vi "DAQ_Torque_Cell.vi"(6 "stop 2":bool) -> ()   [LabVIEW 2020]
doc: "I. Description:\nThis example demonstrates how to continuously acquire data (Waveform) using the DAQ device's internal clock and an analog slope start trigger.\n\nII. Instructions for Running:\n1. Select the physical channel to correspond to where your signal is input on the DAQ device.\n2. Enter the minimum and maximum voltage ranges.\nNote: For better accuracy try to match the Input Ranges to the expected voltage level of the measured signal.\n3. Set the rate of the acquisition. Also set the Samples to Read control. This will determine how many samples are read each time the while loop iterates. This also determines how many points are plotted on the graph each iteration.\nNote: The rate should be at least twice as fast as the maximum frequency component of the signal being acquired.\n4. Set the source of the Analog Slope Start Trigger.\n5. Set the slope and level of desired analog edge condition.\n\nIII. Block Diagram Steps:\n1. Create an analog input voltage channel.\n2. Set the rate for the sample clock. Additionally, define the sample mode to be continuous.\n3. Define the parameters for an Analog Slope Start Trigger.\n4. Call the Start VI to start the acquisition.\n5. Read the waveform data in a loop until the user hits the stop button or an error occurs.\n6. Call the Clear Task VI to clear the Task.\n7. Use the popup dialog box to display an error if any.\n\nIV. I/O Connections Overview:\nMake sure your signal input terminal matches the Physical Channel I/O control. Also, make sure your analog trigger terminal matches the Trigger Source Control. For further connection information, refer to your hardware reference manual."
uses:
  <vilib>/Utility/error.llb/DialogType.ctl
  <vilib>/ULx/Create Channel.llb/ULx Create Channel (AI-Voltage-Basic).vi
  <vilib>/ULx/Timing.llb/ULx Timing (Sample Clock).vi
  <vilib>/ULx/Read.llb/ULx Read (Analog Wfm 1Chan NSamp).vi
panel:
  out "Torque Graph":waveform(dbl)(graph)
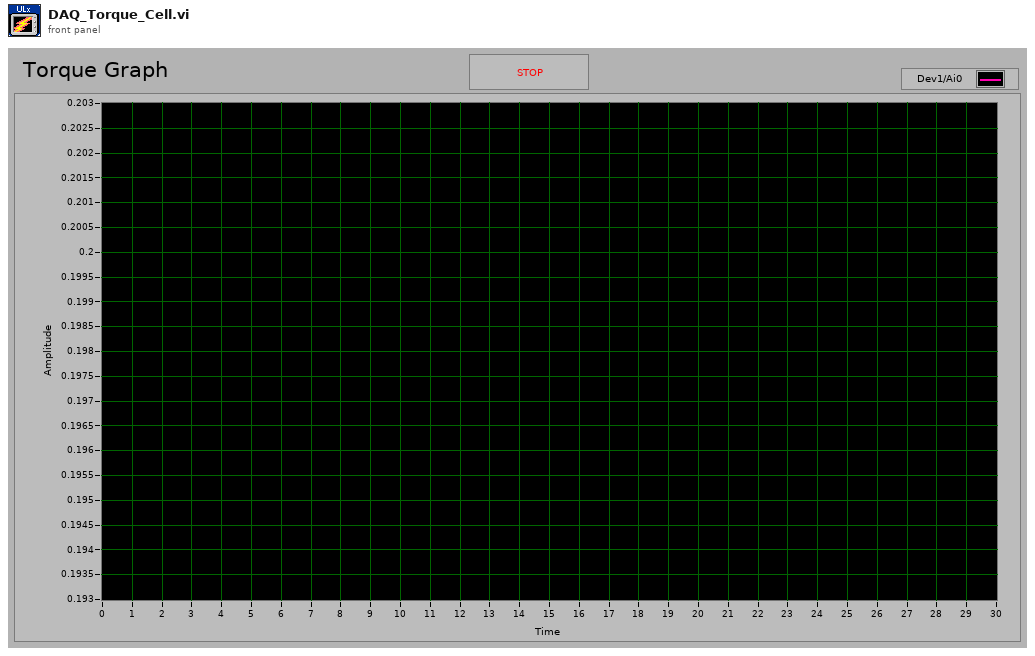
[diagram p1: front panel]
types:
  T1 = typedef "DialogType.ctl" = u16
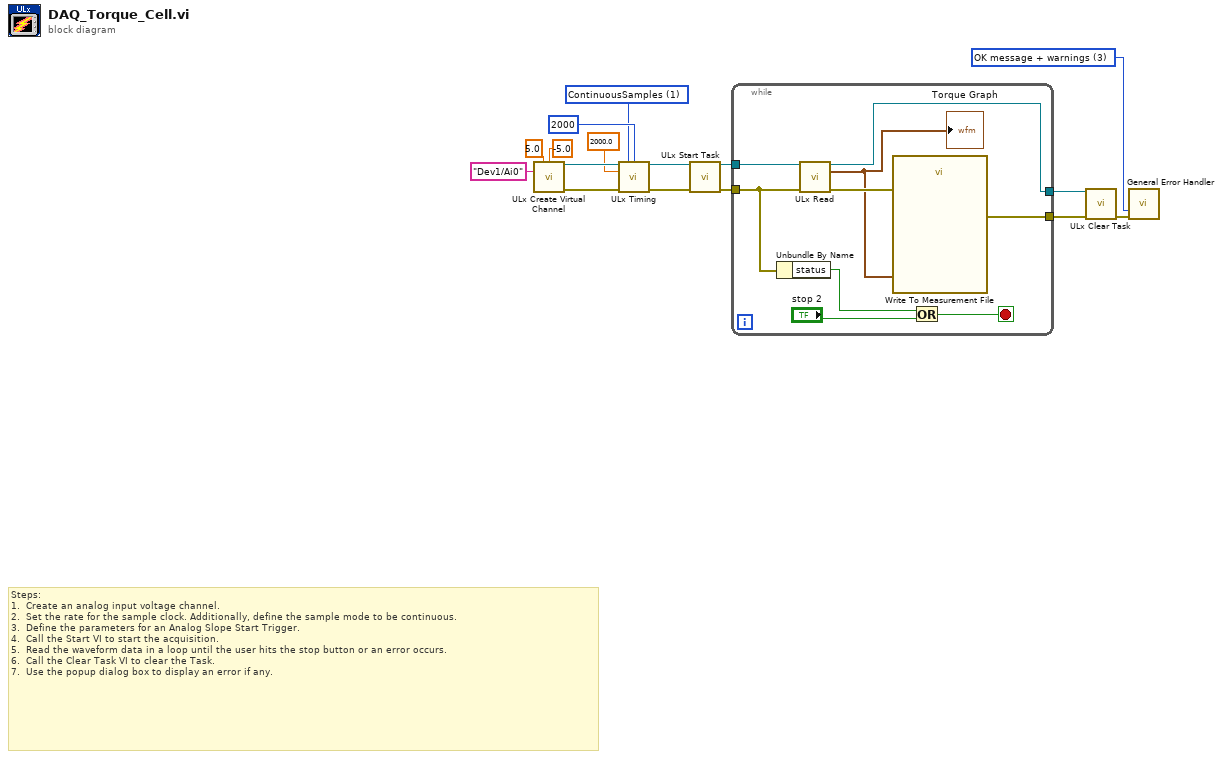
[diagram p0: block diagram]
diagram:
  w5 = 1 items=["FiniteSamples", "ContinuousSamples"] ("sample mode")
  w9 = T1 3 items=["no dialog", "OK message", "continue or stop message", "OK message + warnings", "continue/stop + warnings"] ("type of dialog (OK msg:1)")
  # "Steps: \n1.  Create an analog input voltage channel.\n2.  Set the rate for the sample clock. Additionally, define the sample mode to be continuous.\n3.  Define the parameters for an Analog Slope Start Trigger.\n4.  Call the Start VI to start the acquisition.\n5.  Read the waveform data in a loop until the user hits the stop button or an error occurs.\n6.  Call the Clear Task VI to clear the Task.\n7.  Use the popup dialog box to display an error if any."
  n1 = call-poly <vilib>:"ULx Create Virtual Channel.vi"("maximum value"=5.0, "minimum value"=-5.0, "physical channels"="Dev1/Ai0") -> ("task out"=w13:refnum<k24>, "error out"=w16:errorcluster)  [unwired: 11 in]
  n2 = call-poly <vilib>:"ULx Timing.vi"("task in"=w13, "sample mode"=w5, "samples per channel"=2000, "rate"=2000.0, "error in"=w16) -> ("task out"=w8:refnum<k24>, "error out"=w7:errorcluster)  [unwired: 9 in]
  n3 = call <vilib>:"ULx Start Task.vi"("task in"=w8, "error in"=w7) -> ("task out"=w12:refnum<k24>, "error out"=w15:errorcluster)  [unwired: 12 in]
  n4 = while {
    tunnel: w15 -> [w19]
    tunnel: w12 -> [w25]
    tunnel: [w24] -> w11
    tunnel: [w20] -> w10
    stop <- w22 stop-if-true
    n5 = Unbundle By Name(w19) -> ("status"=w23:bool)
    n6 = call-poly <vilib>:"ULx Read.vi"("task in"=w25, "error in"=w19) -> ("task out"=w24:refnum<k24>, "data"=w17:waveform(dbl), "error out"=w21:errorcluster)  [unwired: 11 in]
    "Torque Graph" <- w17
    n7 = call "Write To Measurement File"("Signals"=w17, "error in (no error)"=w21) -> ("error out"=w20:errorcluster)  [unwired: 15 in, 2 out]
    n8 = Or(x=w23, y="stop 2") -> (x .or. y?=w22:bool)
  }
  n9 = call <vilib>:"ULx Clear Task.vi"("task in"=w11, "error in"=w10) -> ("error out"=w14:errorcluster)  [unwired: 13 in]
  n10 = call <vilib>:"General Error Handler.vi"("type of dialog (OK msg:1)"=w9, "error in (no error)"=w14) -> ()  [unwired: 9 in, 5 out]
